vi "Read Receive Data.vi"(8 "error in (no error)":errorcluster, 11 "NodeRed-LV-Interface in":refnum<class "NodeRed-LV-Interface.lvclass">) -> (0 "error out":errorcluster, 2 "Receive data":refnum<user-event>, 3 "NodeRed-LV-Interface out":refnum<class "NodeRed-LV-Interface.lvclass">)   [LabVIEW 2020, in "NodeRed-LV-Interface.lvclass"]
uses:
  NodeRed-LV-Interface.lvclass
  NodeRed-LV-Interface.lvclass/NodeRed-LV-Interface.ctl
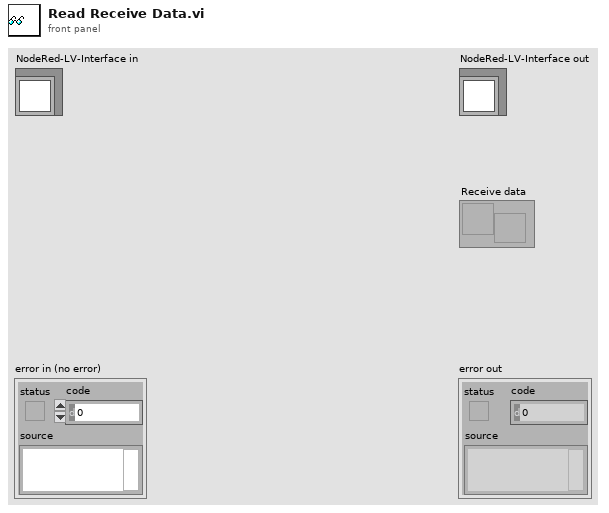
[diagram p1: front panel]
types:
  T1 = cluster{"Send data":refnum<user-event>, "Receive data":refnum<user-event>, "UDP Engine":refnum<vi>, "IP Address":string, "Port":u16}
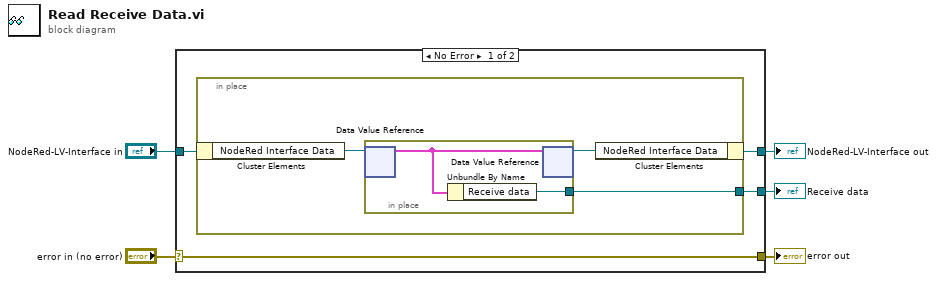
[diagram p0: block diagram]
diagram:
  n1 = case shown="No Error" "error in (no error)" {
    selector: "error in (no error)" -> [w9 w15]
    tunnel: [w9 w15] -> w4
    tunnel: [w7 w16] -> w2
    tunnel: "NodeRed-LV-Interface in" -> [w8 w16]
    tunnel: [w6 _] -> w1
    frame No Error {
      n2 = in-place {
        in-place-border: [w10] -> w6
        n3 = in-place-cluster #1(w8) -> ("NodeRed Interface Data"=w12:refnum<data-value>)
        n4 = in-place {
          in-place-border: [w13] -> w10
          n5 = in-place-dvr #2(w12) -> (w14:T1)  [unwired: 1 out]
          n6 = Unbundle By Name(w14) -> ("Receive data"=w13:refnum<user-event>)
          n7 = in-place-dvr #2(w14) -> (w11:refnum<data-value>)  [unwired: 1 out]
        }
        n8 = in-place-cluster #1("NodeRed Interface Data"=w11) -> (w7:refnum<class "NodeRed-LV-Interface.lvclass">)
      }
    }
    frame Error {
    }
  }
  "error out" <- w4
  "NodeRed-LV-Interface out" <- w2
  "Receive data" <- w1
